vi "TreeDirectory Example.vi"() -> ()   [LabVIEW 2015]
doc: "AA simple example of a QControl. This TreeDirectory QControl loads the directory given in Path to the Tree. The QControl then lets the user open files through double-clicking.\n\n1. Click Run.\n2. Choose a Path. (Large Directories could take a while to load)\n3. Directory will be loaded into Tree.\n4. Double-clicking item will launch/open item.\n5. Click Stop to end program.s\n<b> </b> <b> </b>\n©2016 Q Software Innovations, LLC (QSI)\nwritten by Quentin Alldredge\nproduced in LabVIEW 2015\n\nsupport@qsoftwareinnovations.com\nwww.qsoftwareinnovations.com\n\nAll rights reserved.\n\nRedistribution and use in source and binary forms, with or without modification, are permitted provided that the following conditions are met:\n\n * Redistributions of source code must retain the above copyright notice, this list of conditions and the following disclaimer.\n * Redistributions in binary form must reproduce the above copyright notice, this list of conditions and the following disclaimer in the documentation and/or other materials provided with the distribution.\n * Neither the name of Q Software Innovations, LLC. nor the names of its contributors may be used to endorse or promote products derived from this software without specific prior written permission.\n\nTHIS SOFTWARE IS PROVIDED BY THE COPYRIGHT HOLDERS AND CONTRIBUTORS \"AS IS\" AND ANY EXPRESS OR IMPLIED WARRANTIES, INCLUDING, BUT NOT LIMITED TO, THE IMPLIED WARRANTIES OF MERCHANTABILITY AND FITNESS FOR A PARTICULAR PURPOSE ARE DISCLAIMED. IN NO EVENT SHALL THE COPYRIGHT OWNER OR CONTRIBUTORS BE LIABLE FOR ANY DIRECT, INDIRECT, INCIDENTAL, SPECIAL, EXEMPLARY, OR CONSEQUENTIAL DAMAGES (INCLUDING, BUT NOT LIMITED TO, PROCUREMENT OF SUBSTITUTE GOODS OR SERVICES; LOSS OF USE, DATA, OR PROFITS; OR BUSINESS INTERRUPTION) HOWEVER CAUSED AND ON ANY THEORY OF LIABILITY, WHETHER IN CONTRACT, STRICT LIABILITY, OR TORT (INCLUDING NEGLIGENCE OR OTHERWISE) ARISING IN ANY WAY OUT OF THE USE OF THIS SOFTWARE, EVEN IF ADVISED OF THE POSSIBILITY OF SUCH DAMAGE."
uses:
  QControl Classes/TreeDirectory/TreeDirectory.lvclass
panel:
  in  "Path":path
  in  "Stop Button":bool
  in  "Tree":string(tree)
  # "TreeDirectory QControl Example\n\nA simple example of a QControl.  This TreeDirectory QControl loads the directory given in Path to the Tree.  The QControl then lets the user open files through double-clicking.\n\n1. Click Run.\n2. Choose a Path.  (Large Directories could take a while to load)\n3. Directory will be loaded into Tree.\n4. Double-clicking item will launch/open item.\n5. Click Stop to end program."
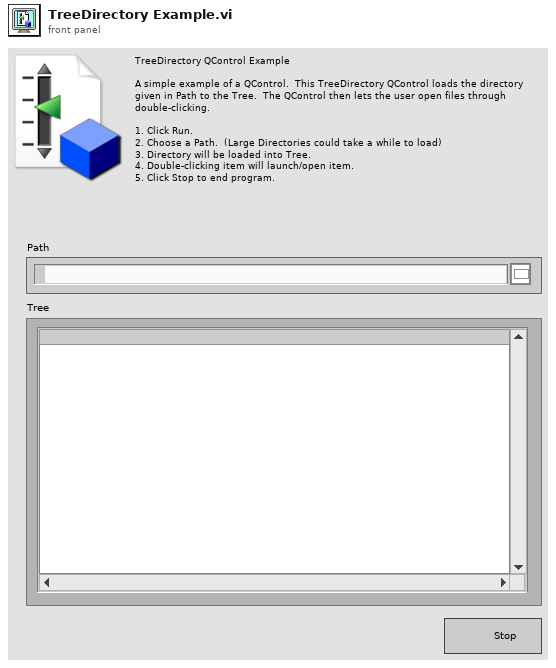
[diagram p1: front panel]
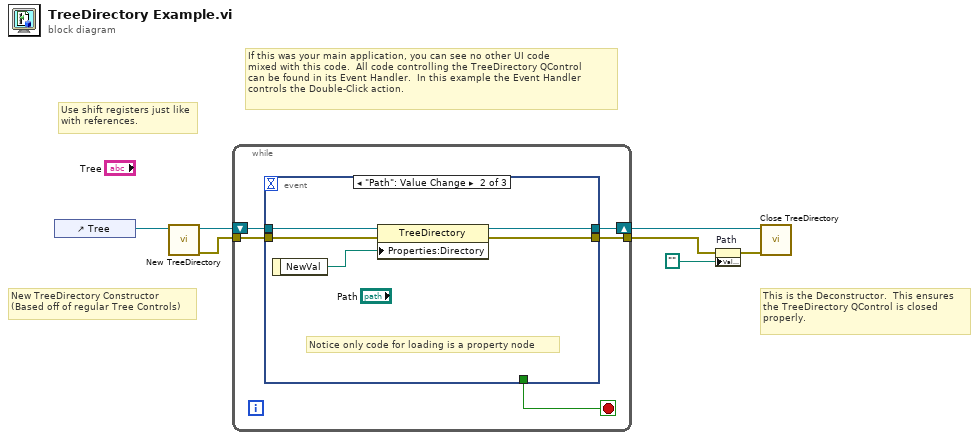
[diagram p0: block diagram]
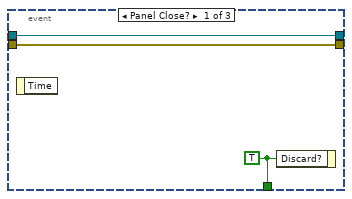
[diagram p2: hidden frame]
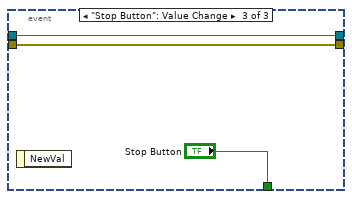
[diagram p3: hidden frame]
diagram:
  # "Use shift registers just like\nwith references."
  # "This is the Deconstructor.  This ensures \nthe TreeDirectory QControl is closed \nproperly."
  # "If this was your main application, you can see no other UI code\nmixed with this code.  All code controlling the TreeDirectory QControl\ncan be found in its Event Handler.  In this example the Event Handler \ncontrols the Double-Click action."
  # "New TreeDirectory Constructor\n(Based off of regular Tree Controls)"
  n1 = control-ref of="Tree"() -> (w6:refnum<vi>)
  n2 = call "New TreeDirectory.vi"("Reference"=w6) -> ("error out"=w4:errorcluster, "TreeDirectory out"=w5:refnum<class "TreeDirectory.lvclass">)  [unwired: 9 in]
  n3 = while {
    tunnel: w4 -> [w9]
    tunnel: [w8] -> w3
    shift-right: [w11] -> w7
    shift-left: w5 -> [w10]
    stop <- w12 stop-if-true
    n4 = event shown="[1] \"Path\": Value Change" {
      selector: _ -> [_ _ _]
      dyn-events: _ -> [_ _ _]
      timeout: _ -> [_ _ _]
      tunnel: [w15 _ "Stop Button"] -> w12
      tunnel: [w14 w18 w22] -> w11
      tunnel: w10 -> [w14 w20 w22]
      tunnel: w9 -> [w13 w17 w21]
      tunnel: [w13 w16 w21] -> w8
      event Panel Close? {
        w15 = TRUE ("Discard?")
        n5 = event-data() -> ()  [unwired: 1 in, 1 out]
        n6 = event-data("Discard?"=w15) -> ()  [unwired: 1 in, 1 out]
      }
      event "Path": Value Change {
        # "Notice only code for loading is a property node"
        n7 = event-data() -> ("NewVal"=w19:path)  [unwired: 1 in]
        n8 = property class="TreeDirectory"(reference=w20, error in=w17, "Properties:Directory"=w19) -> (reference out=w18:refnum<class "TreeDirectory.lvclass">, error out=w16:errorcluster)
      }
      event "Stop Button": Value Change {
        n9 = event-data() -> ()  [unwired: 1 in, 1 out]
      }
    }
  }
  n10 = property on="Path" class="Path"(error in=w3, "Value"=path "") -> (error out=w2:errorcluster)  [unwired: 1 in, 1 out]
  n11 = call "Close TreeDirectory.vi"("error in (no error)"=w2, "TreeDirectory in"=w7) -> ()  [unwired: 8 in, 2 out]
